vi "PropertyChangedEventCallbackForBufferIndex.vi"(4 "?":refnum<vi>, 5 "Event Data":cluster{"sender":refnum<k24>, "e":refnum<k24>}, 6 "Control Ref":refnum<k24>, 7 "Event Common Data":T1) -> ()   [LabVIEW 2018]
uses:
  C:/Users/Public/Documents/Photometrics/PMQI-LabViewSamples/Examples/Dependencies/PVCamNET.dll
  Public/Documents/Photometrics/PMQI-LabViewSamples/Examples/Dependencies/PVCamNET.dll
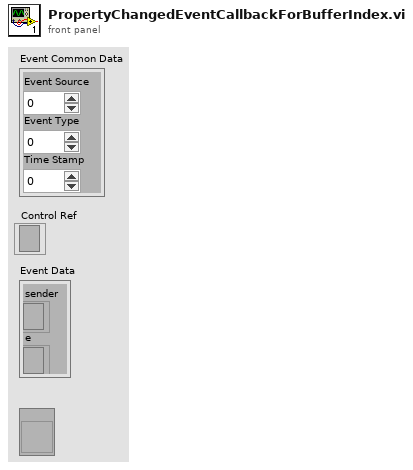
[diagram p1: front panel]
types:
  T1 = cluster{"Event Source":i32, "Event Type":u32, "Time Stamp":u32}
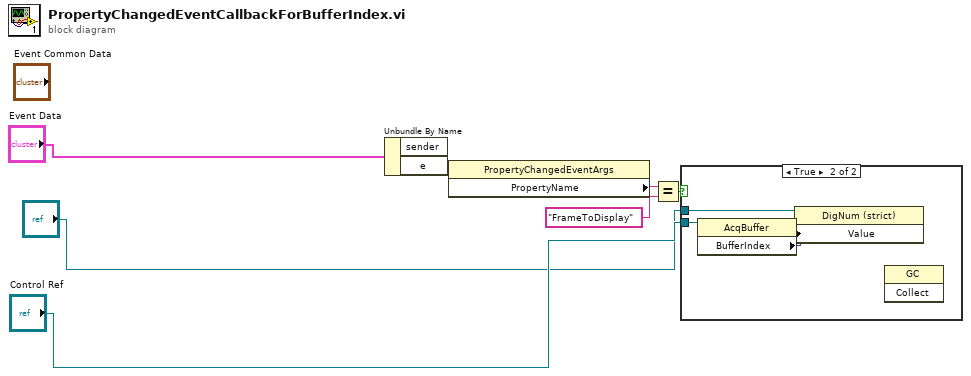
[diagram p0: block diagram]
diagram:
  n1 = Unbundle By Name("Event Data") -> ("e"=w7:refnum<k24>)  [unwired: 1 out]
  n2 = property class="PropertyChangedEventArgs"(reference=w7) -> ("PropertyName"=w6:string)  [unwired: 1 in, 2 out]
  n3 = Equal?(x=w6, y="FrameToDisplay") -> (x = y?=w4:bool)
  n4 = case shown="True" w4 {
    tunnel: "?" -> [_ w10]
    tunnel: "Control Ref" -> [_ w9]
    frame False {
    }
    frame True {
      n5 = property class="AcqBuffer"(reference=w9) -> ("BufferIndex"=w8:i32)  [unwired: 1 in, 2 out]
      n6 = property class="DigNum (strict)"(reference=w10, "Value"=w8) -> ()  [unwired: 1 in, 2 out]
      n7 = invoke class="GC" method="Collect"() -> ()  [unwired: 3 in, 3 out]
    }
  }
